vi "Configure.vi"(8 "error in (no error)":errorcluster, 11 "ConfocalStage in":refnum<class "ConfocalStage.lvclass">) -> (0 "error out":errorcluster, 2 "cancelled?":bool, 3 "ConfocalStage out":refnum<class "ConfocalStage.lvclass">)   [LabVIEW 2012, in "ConfocalStage.lvclass"]
doc: "The configure method configures the details for the RabbitMQ connection, the observers and the mapping script.\n\nIn the derived class, make a call to the parent for setting these parameters."
uses:
  ConfocalStage.lvclass
  <vilib>/Utility/miscctls.llb/LVPointTypeDef.ctl
  ConfocalStage.lvclass/ConfocalStage.ctl
  <vilib>/Distrio/Murmex/Murmex/Murmex.lvclass
panel:
  in  "button:cancel":bool
  in  "button:configure murmex":bool
  in  "button:ok":bool
  in  "Tab Control":enum32{"VISA", "Stages"}(tab)
  in  "stop bits":u16(ring)=20 items=["1.0"=10, "1.5"=15, "2.0"=20]
  in  "flow control":u16(ring) items=["None", "XON/XOFF", "RTS/CTS", "XON/XOFF & RTS/CTS", "DTR/DSR", "XON/XOFF & DTR/DSR"]
  in  "baud rate":u32
  in  "data bits":u16
  in  "send termination char?":bool
  in  "termination char":u8
  in  "parity (0:none)":enum16{"None", "Odd", "Even", "Mark", "Space"}(ring)
  in  "COM port":refnum<visa-resource-name>
  in  "reporting folder":path
  in  "position conversion focus":dbl
  in  "position conversion Y":dbl
  in  "position conversion X":dbl
  in  "speed conversion":dbl
  in  "accelleration ramp":dbl[unit]
  in  "startup speed":dbl[unit]
  # "(CarriageReturn=13)"
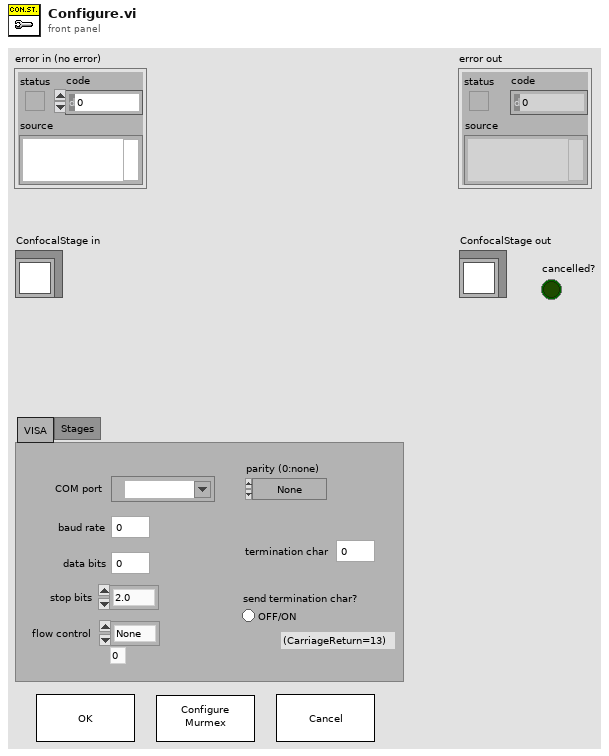
[diagram p1: front panel]
types:
  T1 = typedef "LVPointTypeDef.ctl" = cluster{"Horizontal":i16, "Vertical":i16}
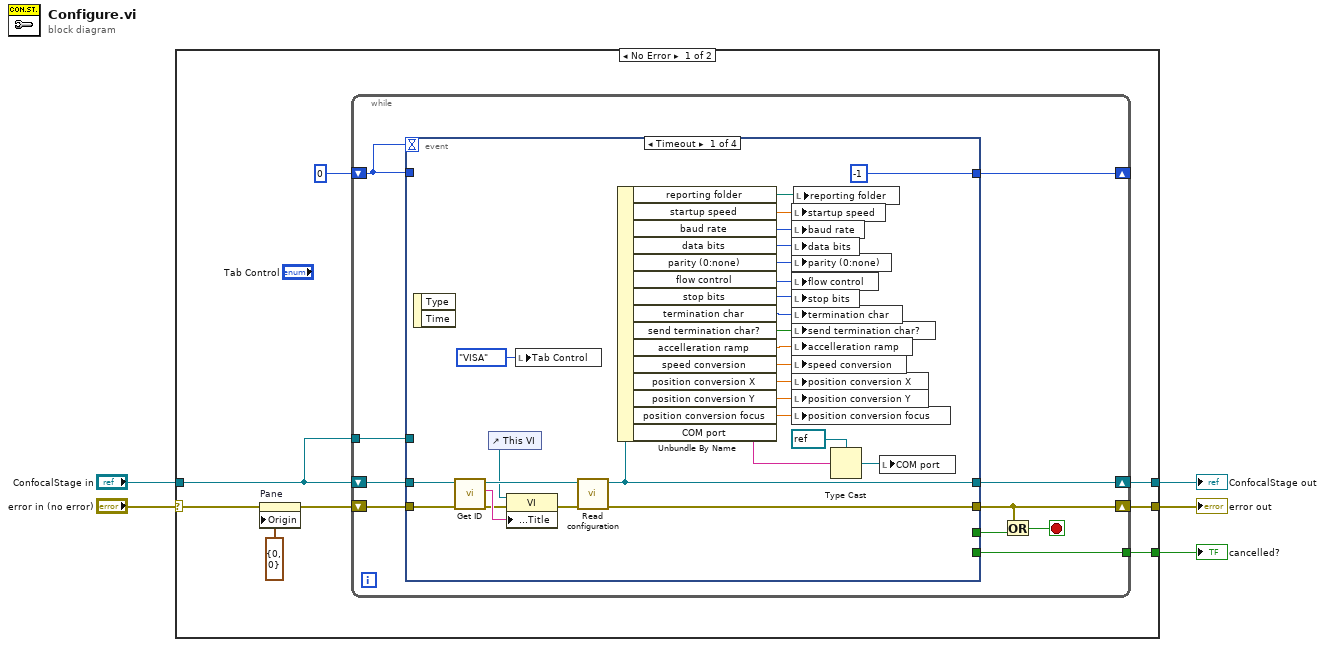
[diagram p0: block diagram]
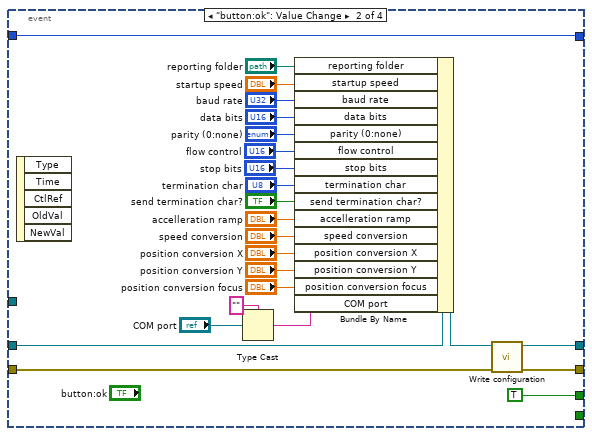
[diagram p2: hidden frame]
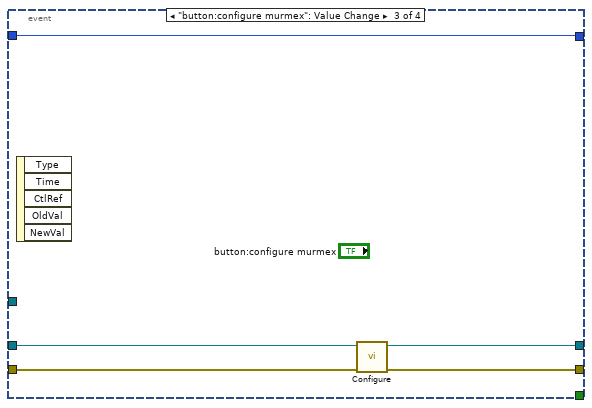
[diagram p3: hidden frame]
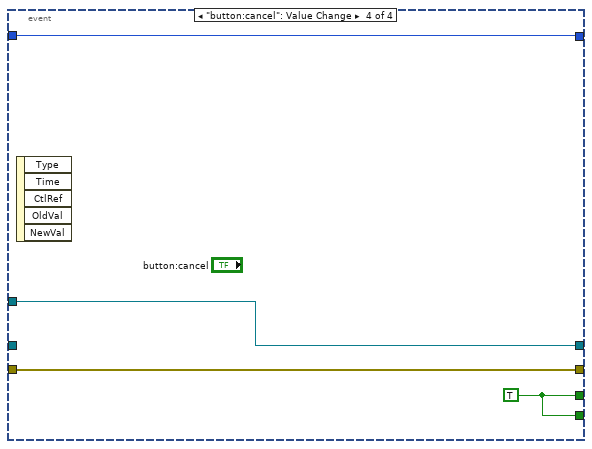
[diagram p4: hidden frame]
diagram:
  n1 = case shown="No Error" "error in (no error)" {
    selector: "error in (no error)" -> [w12 w85]
    tunnel: "ConfocalStage in" -> [w10 w86]
    tunnel: [w8 w85] -> w3
    tunnel: [w7 w86] -> w2
    tunnel: [w6 _] -> w1
    frame No Error {
      n2 = property on="Pane" class="Pane"(error in=w12, "Origin"=T1 {"Horizontal"=0, "Vertical"=0}) -> (error out=w11:errorcluster)  [unwired: 1 in, 1 out]
      n3 = while {
        shift-right: [w21] -> w7
        shift-left: w10 -> [w22]
        shift-right: [w18] -> w8
        shift-left: w11 -> [w23]
        tunnel: w10 -> [w15]
        shift-right: [w20] -> _
        shift-left: 0 -> [w19]
        tunnel: [w14] -> w6
        stop <- w16 stop-if-true
        n4 = event shown="[0] Timeout" {
          selector: _ -> [_ _ _ _]
          dyn-events: _ -> [_ _ _ _]
          timeout: w19 -> [_ _ _ _]
          tunnel: w23 -> [w45 w74 w80 w82]
          tunnel: w22 -> [w44 w71 w79 _]
          tunnel: [w30 w72 w78 w83] -> w21
          tunnel: [-1 w75 w76 w84] -> w20
          tunnel: w19 -> [_ w75 w76 w84]
          tunnel: [w28 w73 w77 w82] -> w18
          tunnel: [_ TRUE _ w81] -> w17
          tunnel: w15 -> [_ _ _ w83]
          tunnel: [_ _ _ w81] -> w14
          event Timeout {
            n5 = event-data() -> ()  [unwired: 1 in, 2 out]
            n6 = call <vilib>:"Get ID.vi"("error in (no error)"=w45, "Murmex in"=w44) -> ("error out"=w46:errorcluster, "component id"=w50:string, "Murmex out"=w49:refnum<class "ConfocalStage.lvclass">)  [unwired: 7 in]
            n7 = control-ref of="This VI"() -> (w47:refnum<vi>)
            n8 = property class="VI"(reference=w47, error in=w46, "Front Panel.Title"=w50) -> (error out=w48:errorcluster)  [unwired: 1 out]
            n9 = local write "Tab Control"(enum32{"VISA", "Stages"}."VISA" ("Tab Control")) -> ()
            n10 = call <vilib>:"Read configuration.vi"("error in (no error)"=w48, "Murmex in"=w49) -> ("error out"=w28:errorcluster, "Murmex out"=w30:refnum<class "ConfocalStage.lvclass">)  [unwired: 7 in, 1 out]
            n11 = Unbundle By Name(w30) -> ("reporting folder"=w24:path, "startup speed"=w43:dbl[unit], "baud rate"=w42:u32, "data bits"=w32:u16, "parity (0:none)"=w39:enum16{"None", "Odd", "Even", "Mark", "Space"}, "flow control"=w38:u16, "stop bits"=w41:u16, "termination char"=w40:u8, "send termination char?"=w31:bool, "accelleration ramp"=w33:dbl[unit], "speed conversion"=w36:dbl, "position conversion X"=w34:dbl, "position conversion Y"=w35:dbl, "position conversion focus"=w37:dbl, "COM port"=w27:string)
            n12 = local write "startup speed"(w43) -> ()
            n13 = local write "baud rate"(w42) -> ()
            n14 = local write "data bits"(w32) -> ()
            n15 = local write "parity (0:none)"(w39) -> ()
            n16 = local write "flow control"(w38) -> ()
            n17 = local write "stop bits"(w41) -> ()
            n18 = local write "termination char"(w40) -> ()
            n19 = local write "send termination char?"(w31) -> ()
            n20 = local write "accelleration ramp"(w33) -> ()
            n21 = local write "speed conversion"(w36) -> ()
            n22 = local write "position conversion X"(w34) -> ()
            n23 = local write "position conversion Y"(w35) -> ()
            n24 = local write "position conversion focus"(w37) -> ()
            n25 = local write "reporting folder"(w24) -> ()
            n26 = Type Cast(type=refnum<visa-resource-name> refnum ("COM port"), x=w27) -> (*(type *) &x=w25:refnum<visa-resource-name>)
            n27 = local write "COM port"(w25) -> ()
          }
          event "button:ok": Value Change {
            n28 = event-data() -> ()  [unwired: 1 in, 5 out]
            n29 = Type Cast(type="" ("configuration.Serial port.COM port"), x="COM port") -> (*(type *) &x=w54:string)
            n30 = Bundle By Name(cluster=w71, "reporting folder"="reporting folder", "startup speed"="startup speed", "baud rate"="baud rate", "data bits"="data bits", "parity (0:none)"="parity (0:none)", "flow control"="flow control", "stop bits"="stop bits", "termination char"="termination char", "send termination char?"="send termination char?", "accelleration ramp"="accelleration ramp", "speed conversion"="speed conversion", "position conversion X"="position conversion X", "position conversion Y"="position conversion Y", "position conversion focus"="position conversion focus", "COM port"=w54) -> (w70:refnum<class "ConfocalStage.lvclass">)
            n31 = call <vilib>:"Write configuration.vi"("error in (no error)"=w74, "Murmex in"=w70) -> ("error out"=w73:errorcluster, "Murmex out"=w72:refnum<class "ConfocalStage.lvclass">)  [unwired: 8 in]
          }
          event "button:configure murmex": Value Change {
            n32 = event-data() -> ()  [unwired: 1 in, 5 out]
            n33 = call-parent "Configure.vi"("error in (no error)"=w80, "Murmex in"=w79) -> ("error out"=w77:errorcluster, "Murmex out"=w78:refnum<class "ConfocalStage.lvclass">)  [unwired: 7 in, 1 out]
          }
          event "button:cancel": Value Change {
            w81 = TRUE
            n34 = event-data() -> ()  [unwired: 1 in, 5 out]
          }
        }
        n35 = Or(x=w18, y=w17) -> (x .or. y?=w16:bool)
      }
    }
    frame Error {
    }
  }
  "error out" <- w3
  "ConfocalStage out" <- w2
  "cancelled?" <- w1
